vi "lfield_read_saved_experiments.vi"(8 "error in (no error)":errorcluster, 11 "lightfield_class in":refnum<class "lightfield_class.lvclass">) -> (0 "error out":errorcluster, 2 "Saved Experiments":string[](array[string]), 3 "lightfield_class out":refnum<class "lightfield_class.lvclass">)   [LabVIEW 2015, in "lightfield_class.lvclass"]
uses:
  lightfield_class.lvclass
  lightfield_class.lvclass/lightfield_class.ctl
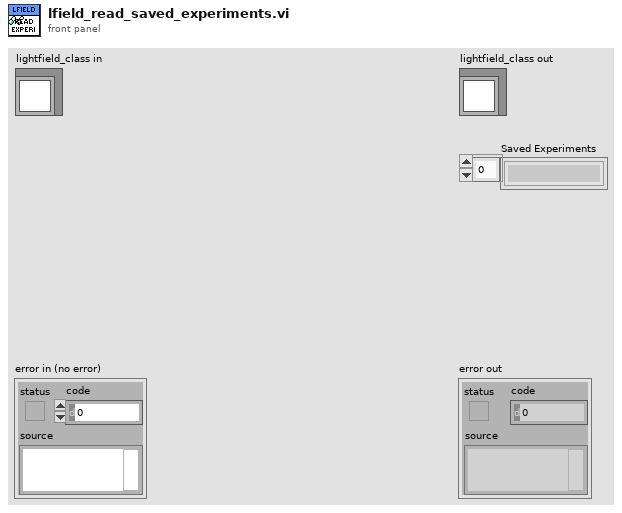
[diagram p1: front panel]
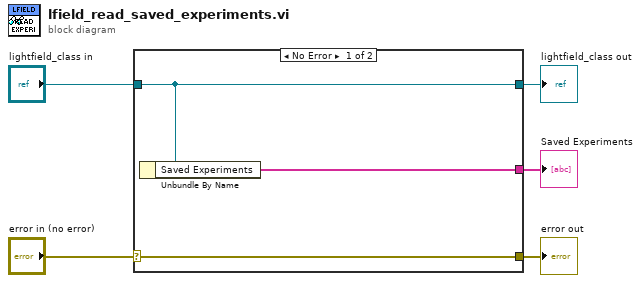
[diagram p0: block diagram]
diagram:
  n1 = case shown="No Error" "error in (no error)" {
    selector: "error in (no error)" -> [w8 w9]
    tunnel: [w8 w9] -> w4
    tunnel: [w7 w10] -> w2
    tunnel: "lightfield_class in" -> [w7 w10]
    tunnel: [w6 _] -> w1
    frame No Error {
      n2 = Unbundle By Name(w7) -> ("Saved Experiments"=w6:string[])
    }
    frame Error {
    }
  }
  "error out" <- w4
  "lightfield_class out" <- w2
  "Saved Experiments" <- w1
